vi "getValueList.vi"(8 "error in (no error)":errorcluster, 11 "node in":refnum<class "node.lvclass">) -> (0 "error out":errorcluster, 2 "Array":dbl[](array[numeric]), 3 "node out":refnum<class "node.lvclass">)   [LabVIEW 2014, in "Linked List.lvlib" / "node.lvclass"]
uses:
  node.lvclass
  node.lvclass/node.ctl
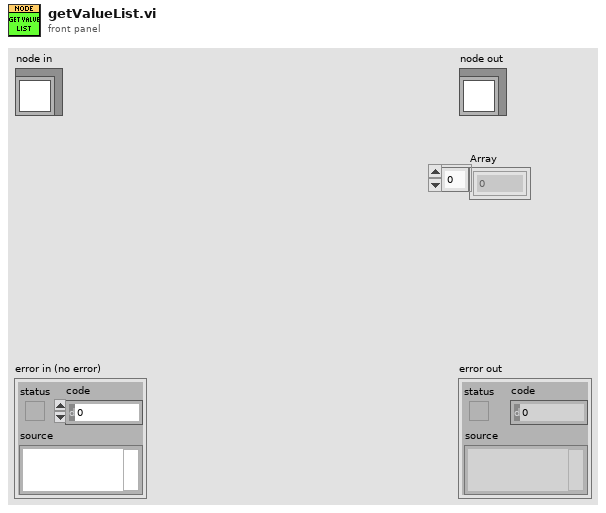
[diagram p1: front panel]
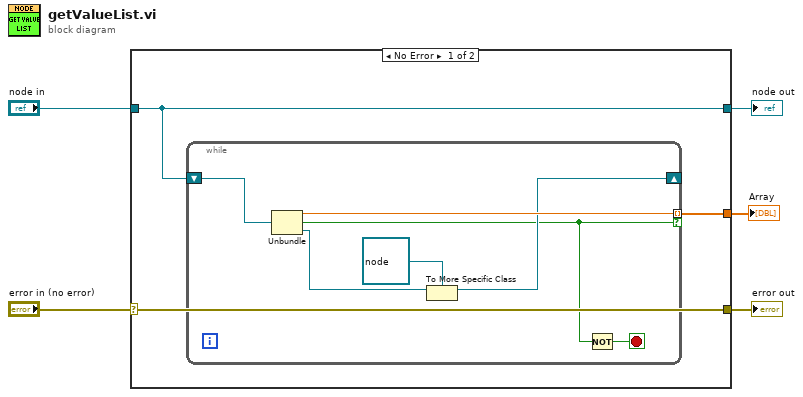
[diagram p0: block diagram]
diagram:
  n1 = case shown="No Error" "error in (no error)" {
    selector: "error in (no error)" -> [w8 w17]
    tunnel: [w8 w17] -> w4
    tunnel: [w7 w16] -> w2
    tunnel: "node in" -> [w7 w16]
    tunnel: [w6 _] -> w1
    frame No Error {
      n2 = while {
        shift-right: [w12] -> _
        shift-left: w7 -> [w15]
        tunnel: [w14] -> w6 mode=indexing if=w10
        stop <- w9 stop-if-true
        n3 = Unbundle(w15) -> (w14:dbl, w10:bool, w13:refnum<class "base.lvclass">)
        n4 = To More Specific Class(target class=refnum<class "node.lvclass"> refnum ("Linked List.lvlib:node"), reference=w13) -> (specific class reference=w12:refnum<class "node.lvclass">)  [unwired: 1 in, 1 out]
        n5 = Not(x=w10) -> (.not. x?=w9:bool)
      }
    }
    frame Error {
    }
  }
  "error out" <- w4
  "node out" <- w2
  "Array" <- w1
